vi "EvaluateDataFlowBlock.vi"(8 "error in (no error)":errorcluster, 9 "data":T2, 10 "config":T1, 11 "Qbus":refnum<class "Qbus.lvclass">) -> (0 "error out":errorcluster, 2 "config":T1)   [LabVIEW 2017, in "McsaDataEventCreator.lvlib"]
uses:
  <vilib>/addons/InsightCM/Devices/Shared/Mcsa/McsaDataEventCreator/McsaDataEventCreator.lvlib
  <vilib>/addons/PointValueMap/PointValueMap.lvlib
  <vilib>/addons/PointValueMap/subVIs/Point_Read_string.vi
  <vilib>/addons/PointValueMap/controls/PointMap.ctl
  <vilib>/addons/InsightCM/Devices/Shared/Common/DVRBuffer/controls/BufferLocation.ctl
  <vilib>/addons/InsightCM/Devices/Shared/Common/DVRBuffer/DVRBuffer.lvlib
  <vilib>/addons/InsightCM/Devices/Shared/Common/DataAccumulator/controls/accumulationType.ctl
  <vilib>/addons/InsightCM/Devices/Shared/Common/DataAccumulator/DataAccumulator.lvlib
  <vilib>/addons/InsightCM/Devices/Shared/Common/DataAccumulator/controls/AccumulationSettings.ctl
  <vilib>/addons/InsightCM/Devices/Shared/Common/DataEventCreator/controls/Reason.ctl
  <vilib>/addons/InsightCM/Devices/Shared/Common/DataEventCreator/DataEventCreator.lvlib
  <vilib>/addons/InsightCM/Devices/Shared/Mcsa/McsaDataEventCreator/controls/AcqParams.ctl
  <vilib>/addons/InsightCM/Devices/Shared/Mcsa/McsaDataEventCreator/controls/DataEventConfig.ctl
  <vilib>/addons/InsightCM/Devices/Shared/Common/DataFlow/DataFlow.lvlib
  <vilib>/addons/InsightCM/Utilities/DataAccessors/controls/wfmSGL_DVR.ctl
  <vilib>/addons/InsightCM/Devices/Shared/Common/DataFlow/controls/Data.ctl
  <vilib>/addons/Qbus/Qbus.lvclass
  <vilib>/addons/InsightCM/Devices/Shared/Mcsa/McsaDataEventCreator/controls/config.ctl
  <vilib>/addons/InsightCM/Devices/Shared/Common/DataFlow/controls/Type.ctl
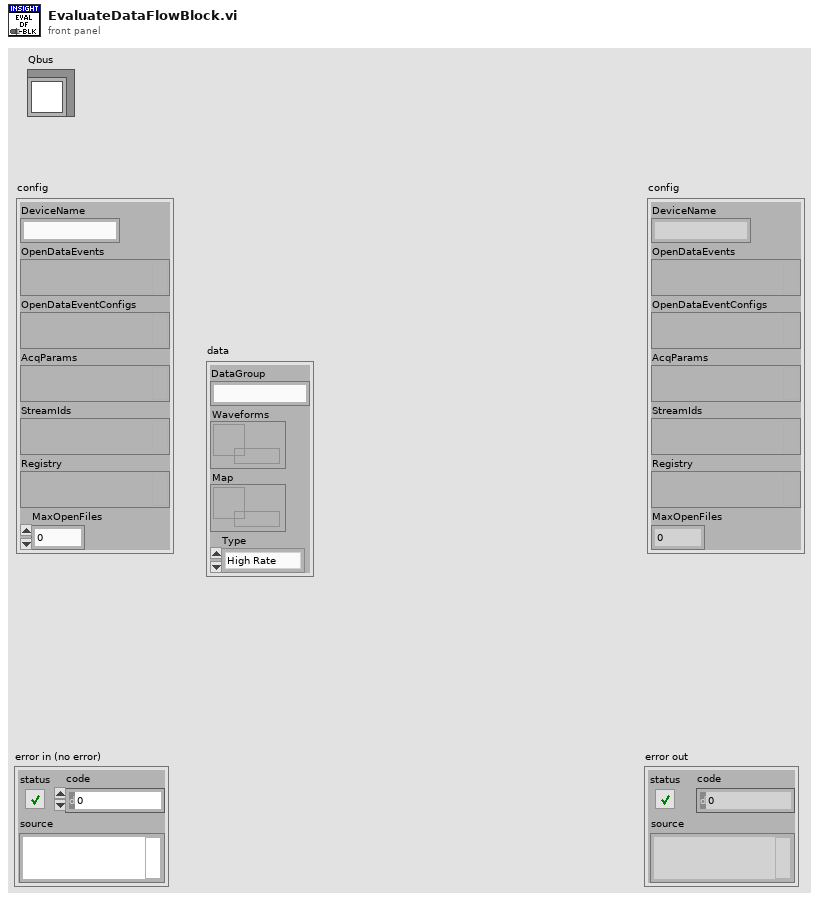
[diagram p1: front panel]
types:
  T1 = typedef "McsaDataEventCreator.lvlib/config.ctl" = cluster{"DeviceName":string, "OpenDataEvents":variant, "OpenDataEventConfigs":variant, "AcqParams":variant, "StreamIds":variant, "Registry":variant, "MaxOpenFiles":i32}
  T2 = typedef "DataFlow.lvlib/Data.ctl" = cluster{"DataGroup":string, "Waveforms":T3, "Map":T4, "Type":T5}
  T3 = typedef "wfmSGL_DVR.ctl" = refnum<data-value>
  T4 = typedef "PointValueMap.lvlib/PointMap.ctl" = refnum<data-value>
  T5 = typedef "DataFlow.lvlib/Type.ctl" = enum16{"High Rate", "Low Rate", "Burst Mode"}
  T6 = typedef "McsaDataEventCreator.lvlib/AcqParams.ctl" = cluster{"Stream":bool, "PreTrigger":i32, "CollectOnEnter":bool, "Enter PreTrigger":i32, "Enter Length":dbl, "CollectOnExit":bool, "ContinuousData":bool, "Accumulation Settings":T7}
  T7 = typedef "DataAccumulator.lvlib/AccumulationSettings.ctl" = cluster{"Type":T8, "Length":dbl, "Max Time (sec)":dbl, "Start Block":T9, "Acquired (sec)":dbl, "Acquired (pulses)":i32, "Initial Pulse Offset":dbl, "Stop Block":T9, "LastBlockAdded":u32}
  T8 = typedef "DataAccumulator.lvlib/accumulationType.ctl" = enum16{"none", "seconds", "revolutions"}
  T9 = typedef "DVRBuffer.lvlib/BufferLocation.ctl" = cluster{"Block":u32, "Index":i32}
  T10 = typedef "DataEventCreator.lvlib/Reason.ctl" = enum16{"Periodic Event", "Delta EU Event", "Trend Event", "Alarm Event", "User Event", "Enter Operating State", "Exit Operating State", "Multiple Events", "Other"}
  T11 = typedef "McsaDataEventCreator.lvlib/DataEventConfig.ctl" = cluster{"AcqParams":T6, "OpState":string, "ExitOpState":bool, "Reason":string, "StreamId":string, "Map":T4, "DataSetIds":variant, "IncludeWaveforms":bool, "TrendPointsOnly":bool}
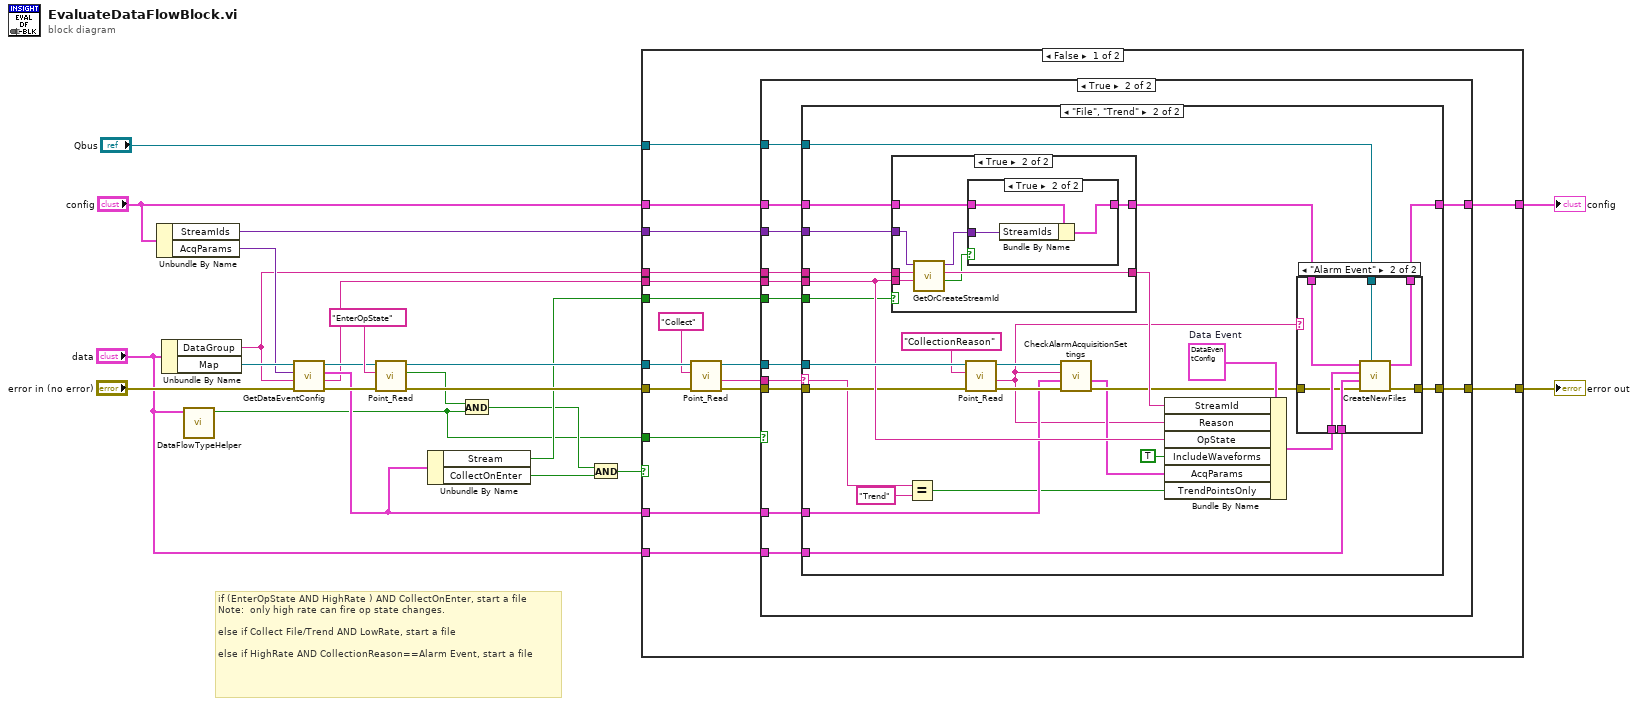
[diagram p0: block diagram]
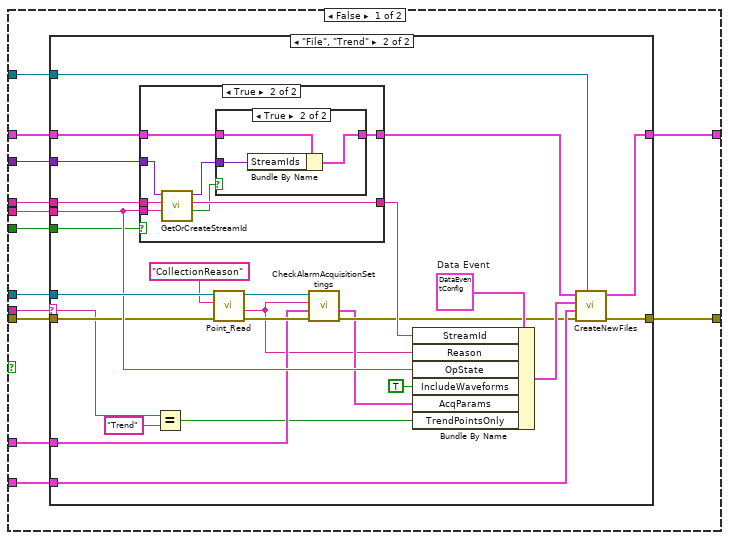
[diagram p2: hidden frame]
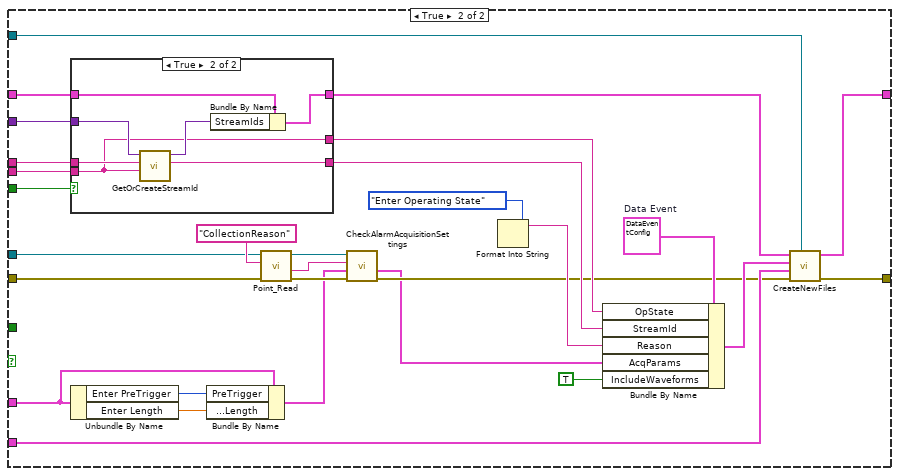
[diagram p10: hidden frame]
diagram:
  # "if (EnterOpState AND HighRate ) AND CollectOnEnter, start a file\nNote:  only high rate can fire op state changes.\n\nelse if Collect File/Trend AND LowRate, start a file\n\nelse if HighRate AND CollectionReason==Alarm Event, start a file"
  n1 = Unbundle By Name("config") -> ("StreamIds"=w21:variant, "AcqParams"=w17:variant)
  n2 = Unbundle By Name("data") -> ("DataGroup"=w16:string, "Map"=w18:T4)
  n3 = call <vilib>:"DataFlowTypeHelper.vi"("data"="data") -> ("high rate"=w2:bool)  [unwired: 8 in, 2 out]
  n4 = call <vilib>:"GetDataEventConfig.vi"("error in (no error)"="error in (no error)", "DataGroup"=w16, "AcqParams"=w17, "map in"=w18) -> ("error out"=w14:errorcluster, "OpState"=w11:string, "acq params"=w12:T6, "map out"=w13:T4)  [unwired: 4 in]
  n5 = call-poly <vilib>:"Point_Read.vi"("Error In"=w14, "Tag"="EnterOpState", "Map"=w13) -> ("Error Out"=w10:errorcluster, "Found?"=w4:bool, "Map Out"=w8:T4)  [unwired: 3 in, 3 out]
  n6 = Unbundle By Name(w12) -> ("Stream"=w5:bool, "CollectOnEnter"=w7:bool)
  n7 = And(x=w4, y=w2) -> (x .and. y?=w3:bool)
  n8 = And(x=w3, y=w7) -> (x .and. y?=w6:bool)
  n9 = case shown="False" w6 {
    tunnel: [w40 w181] -> w22
    tunnel: w21 -> [w39 w186]
    tunnel: "config" -> [w36 w185]
    tunnel: [w33 w178] -> w19
    tunnel: w16 -> [w32 w184]
    tunnel: w12 -> [w37 w166]
    tunnel: w11 -> [w38 w176]
    tunnel: w10 -> [w29 w164]
    tunnel: "data" -> [w34 w180]
    tunnel: "Qbus" -> [w35 w177]
    tunnel: w8 -> [w28 w165]
    tunnel: w5 -> [w31 w171]
    tunnel: w2 -> [w24 _]
    frame False {
      n10 = call-poly <vilib>:"Point_Read.vi"("Error In"=w29, "Tag"="Collect", "Map"=w28) -> ("Error Out"=w30:errorcluster, "Value"=w25:string, "Map Out"=w27:T4)  [unwired: 3 in, 3 out]
      n11 = case shown="True" w24 {
        tunnel: [w53 w107] -> w40
        tunnel: w39 -> [w52 w106]
        tunnel: w38 -> [w51 w105]
        tunnel: w37 -> [w50 w104]
        tunnel: w36 -> [w49 w103]
        tunnel: w35 -> [w48 w102]
        tunnel: w34 -> [w47 w101]
        tunnel: [w46 w100] -> w33
        tunnel: w32 -> [w45 w99]
        tunnel: w31 -> [w44 w98]
        tunnel: w30 -> [w43 w97]
        tunnel: w27 -> [w42 w96]
        tunnel: w25 -> [w41 w95]
        frame False {
          n12 = case shown="\"File\", \"Trend\"" w41 {
            selector: w41 -> [_ w57]
            tunnel: w42 -> [_ w81]
            tunnel: w43 -> [w54 w70]
            tunnel: [w54 w76] -> w53
            tunnel: w52 -> [_ w73]
            tunnel: w51 -> [_ w71]
            tunnel: w50 -> [_ w61]
            tunnel: w49 -> [w55 w67]
            tunnel: w48 -> [_ w79]
            tunnel: w47 -> [_ w77]
            tunnel: [w55 w75] -> w46
            tunnel: w45 -> [_ w72]
            tunnel: w44 -> [_ w69]
            frame Default {
            }
            frame "File", "Trend" {
              w65 = T11 {"AcqParams"={"Stream"=FALSE, "PreTrigger"=0, "CollectOnEnter"=FALSE, "Enter PreTrigger"=0, "Enter Length"=0.0, "CollectOnExit"=FALSE, "ContinuousData"=FALSE, "Accumulation Settings"={"Type"=enum."none", "Length"=0.0, "Max Time (sec)"=0.0, "Start Block"={"Block"=0, "Index"=0}, "Acquired (sec)"=0.0, "Acquired (pulses)"=0, "Initial Pulse Offset"=0.0, "Stop Block"={"Block"=0, "Index"=0}, "LastBlockAdded"=0}}, "OpState"="", "ExitOpState"=FALSE, "Reason"="", "StreamId"="", "Map"=refnum, "DataSetIds"=variant, "IncludeWaveforms"=FALSE, "TrendPointsOnly"=FALSE}  # Data Event
              n13 = case shown="True" w69 {
                tunnel: w73 -> [_ w90]
                tunnel: w72 -> [_ w89]
                tunnel: w71 -> [_ w88]
                tunnel: [_ w87] -> w68
                tunnel: w67 -> [w82 w85]
                tunnel: [w82 w84] -> w66
                frame False {
                }
                frame True {
                  n14 = call <vilib>:"GetOrCreateStreamId.vi"("operating state"=w88, "data group"=w89, "stream Ids"=w90) -> ("new streamId"=w83:bool, "stream id"=w87:string, "streamIds out"=w86:variant)  [unwired: 5 in, 1 out]
                  n15 = case shown="True" w83 {
                    tunnel: w86 -> [_ w94]
                    tunnel: w85 -> [w91 w93]
                    tunnel: [w91 w92] -> w84
                    frame False {
                    }
                    frame True {
                      n16 = Bundle By Name(cluster=w93, "StreamIds"=w94) -> (w92:T1)
                    }
                  }
                }
              }
              n17 = Equal?(x=w57, y="Trend") -> (x = y?=w58:bool)
              n18 = call-poly <vilib>:"Point_Read.vi"("Error In"=w70, "Tag"="CollectionReason", "Map"=w81) -> ("Error Out"=w64:errorcluster, "Value"=w56:string, "Map Out"=w62:T4)  [unwired: 3 in, 3 out]
              n19 = call <vilib>:"CheckAlarmAcquisitionSettings.vi"("error in (no error)"=w64, "acq config in"=w61, "collection reason"=w56, "map"=w62) -> ("error out"=w63:errorcluster, "acq config out"=w60:T6)  [unwired: 6 in]
              n20 = Bundle By Name(cluster=w65, "StreamId"=w68, "Reason"=w56, "OpState"=w71, "IncludeWaveforms"=TRUE, "AcqParams"=w60, "TrendPointsOnly"=w58) -> (w78:T11)
              n21 = call <vilib>:"CreateNewFiles.vi"("Qbus"=w79, "error in (no error)"=w63, "data flow"=w77, "data event config"=w78, "config"=w66) -> ("error out"=w76:errorcluster, "config out"=w75:T1)  [unwired: 5 in]
            }
          }
        }
        frame True {
          n22 = case shown="\"File\", \"Trend\"" w95 {
            selector: w95 -> [_ w111]
            tunnel: w96 -> [_ w135]
            tunnel: w97 -> [w108 w124]
            tunnel: [w108 w130] -> w107
            tunnel: w106 -> [_ w127]
            tunnel: w105 -> [_ w125]
            tunnel: w104 -> [_ w115]
            tunnel: w103 -> [w109 w121]
            tunnel: w102 -> [_ w133]
            tunnel: w101 -> [_ w131]
            tunnel: [w109 w129] -> w100
            tunnel: w99 -> [_ w126]
            tunnel: w98 -> [_ w123]
            frame Default {
            }
            frame "File", "Trend" {
              w119 = T11 {"AcqParams"={"Stream"=FALSE, "PreTrigger"=0, "CollectOnEnter"=FALSE, "Enter PreTrigger"=0, "Enter Length"=0.0, "CollectOnExit"=FALSE, "ContinuousData"=FALSE, "Accumulation Settings"={"Type"=enum."none", "Length"=0.0, "Max Time (sec)"=0.0, "Start Block"={"Block"=0, "Index"=0}, "Acquired (sec)"=0.0, "Acquired (pulses)"=0, "Initial Pulse Offset"=0.0, "Stop Block"={"Block"=0, "Index"=0}, "LastBlockAdded"=0}}, "OpState"="", "ExitOpState"=FALSE, "Reason"="", "StreamId"="", "Map"=refnum, "DataSetIds"=variant, "IncludeWaveforms"=FALSE, "TrendPointsOnly"=FALSE}  # Data Event
              n23 = case shown="True" w123 {
                tunnel: w127 -> [_ w153]
                tunnel: w126 -> [_ w152]
                tunnel: w125 -> [_ w151]
                tunnel: [_ w150] -> w122
                tunnel: w121 -> [w145 w148]
                tunnel: [w145 w147] -> w120
                frame False {
                }
                frame True {
                  n24 = call <vilib>:"GetOrCreateStreamId.vi"("operating state"=w151, "data group"=w152, "stream Ids"=w153) -> ("new streamId"=w146:bool, "stream id"=w150:string, "streamIds out"=w149:variant)  [unwired: 5 in, 1 out]
                  n25 = case shown="True" w146 {
                    tunnel: w149 -> [_ w157]
                    tunnel: w148 -> [w154 w156]
                    tunnel: [w154 w155] -> w147
                    frame False {
                    }
                    frame True {
                      n26 = Bundle By Name(cluster=w156, "StreamIds"=w157) -> (w155:T1)
                    }
                  }
                }
              }
              n27 = Equal?(x=w111, y="Trend") -> (x = y?=w112:bool)
              n28 = call-poly <vilib>:"Point_Read.vi"("Error In"=w124, "Tag"="CollectionReason", "Map"=w135) -> ("Error Out"=w118:errorcluster, "Value"=w110:string, "Map Out"=w116:T4)  [unwired: 3 in, 3 out]
              n29 = call <vilib>:"CheckAlarmAcquisitionSettings.vi"("error in (no error)"=w118, "acq config in"=w115, "collection reason"=w110, "map"=w116) -> ("error out"=w117:errorcluster, "acq config out"=w114:T6)  [unwired: 6 in]
              n30 = Bundle By Name(cluster=w119, "StreamId"=w122, "Reason"=w110, "OpState"=w125, "IncludeWaveforms"=TRUE, "AcqParams"=w114, "TrendPointsOnly"=w112) -> (w132:T11)
              n31 = case shown="\"Alarm Event\"" w110 {
                tunnel: w133 -> [_ w144]
                tunnel: w132 -> [_ w143]
                tunnel: w131 -> [_ w142]
                tunnel: [w136 w141] -> w130
                tunnel: [w137 w140] -> w129
                tunnel: w120 -> [w137 w139]
                tunnel: w117 -> [w136 w138]
                frame Default {
                }
                frame "Alarm Event" {
                  n32 = call <vilib>:"CreateNewFiles.vi"("Qbus"=w144, "error in (no error)"=w138, "data flow"=w142, "data event config"=w143, "config"=w139) -> ("error out"=w141:errorcluster, "config out"=w140:T1)  [unwired: 5 in]
                }
              }
            }
          }
        }
      }
    }
    frame True {
      w172 = T11 {"AcqParams"={"Stream"=FALSE, "PreTrigger"=0, "CollectOnEnter"=FALSE, "Enter PreTrigger"=0, "Enter Length"=0.0, "CollectOnExit"=FALSE, "ContinuousData"=FALSE, "Accumulation Settings"={"Type"=enum."none", "Length"=0.0, "Max Time (sec)"=0.0, "Start Block"={"Block"=0, "Index"=0}, "Acquired (sec)"=0.0, "Acquired (pulses)"=0, "Initial Pulse Offset"=0.0, "Stop Block"={"Block"=0, "Index"=0}, "LastBlockAdded"=0}}, "OpState"="", "ExitOpState"=FALSE, "Reason"="", "StreamId"="", "Map"=refnum, "DataSetIds"=variant, "IncludeWaveforms"=FALSE, "TrendPointsOnly"=FALSE}  # Data Event
      n33 = case shown="True" w171 {
        tunnel: w186 -> [_ w195]
        tunnel: w185 -> [w188 w194]
        tunnel: w184 -> [_ w192]
        tunnel: [_ w191] -> w183
        tunnel: w176 -> [w187 w189]
        tunnel: [w188 w190] -> w173
        tunnel: [w187 w189] -> w170
        frame False {
        }
        frame True {
          n34 = call <vilib>:"GetOrCreateStreamId.vi"("operating state"=w189, "data group"=w192, "stream Ids"=w195) -> ("stream id"=w191:string, "streamIds out"=w193:variant)  [unwired: 5 in, 2 out]
          n35 = Bundle By Name(cluster=w194, "StreamIds"=w193) -> (w190:T1)
        }
      }
      n36 = Unbundle By Name(w166) -> ("Enter PreTrigger"=w168:i32, "Enter Length"=w169:dbl)
      n37 = Bundle By Name(cluster=w166, "PreTrigger"=w168, "Accumulation Settings.Length"=w169) -> (w160:T6)
      n38 = call-poly <vilib>:"Point_Read.vi"("Error In"=w164, "Tag"="CollectionReason", "Map"=w165) -> ("Error Out"=w163:errorcluster, "Value"=w161:string, "Map Out"=w162:T4)  [unwired: 3 in, 3 out]
      n39 = call <vilib>:"CheckAlarmAcquisitionSettings.vi"("error in (no error)"=w163, "acq config in"=w160, "collection reason"=w161, "map"=w162) -> ("error out"=w159:errorcluster, "acq config out"=w158:T6)  [unwired: 6 in]
      n40 = Format Into String(Reason."Enter Operating State" ("Reason")) -> (resulting string=w182:string)  [unwired: 3 in, 1 out]
      n41 = Bundle By Name(cluster=w172, "OpState"=w170, "StreamId"=w183, "Reason"=w182, "AcqParams"=w158, "IncludeWaveforms"=TRUE) -> (w179:T11)
      n42 = call <vilib>:"CreateNewFiles.vi"("Qbus"=w177, "error in (no error)"=w159, "data flow"=w180, "data event config"=w179, "config"=w173) -> ("error out"=w181:errorcluster, "config out"=w178:T1)  [unwired: 5 in]
    }
  }
  "error out" <- w22
  "config" <- w19
